vi "varint.vi"() -> ()   [LabVIEW 2011]
panel:
  out "data":i32[](array[numeric])
  out "value 2":variant
  out "value":variant
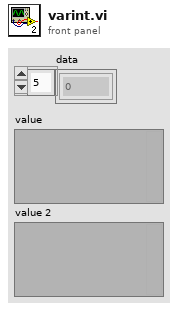
[diagram p1: front panel]
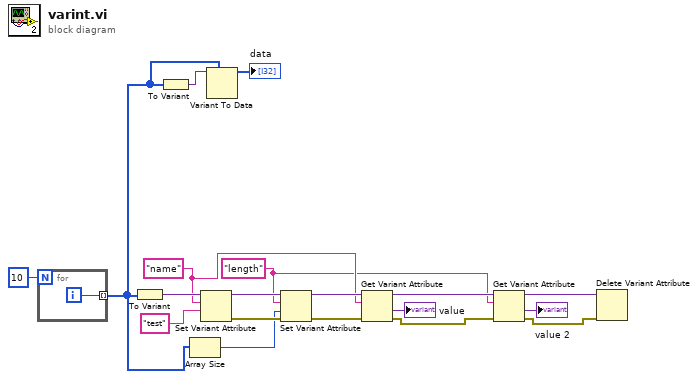
[diagram p0: block diagram]
diagram:
  w7 = "length" ("name")
  w11 = "name" ("name")
  n1 = for {
    N: 10 -> [_]
    tunnel: [w20] -> w2 mode=indexing
    i -> [w20]
  }
  n2 = To Variant(anything=w2) -> (Variant=w18:variant)
  n3 = To Variant(anything=w2) -> (Variant=w3:variant)
  n4 = Array Size(array=w2) -> (size(s)=w14:i32)
  n5 = Set Variant Attribute(Variant=w18, name=w11, value="test" ("name")) -> (Variant out=w16:variant, error out=w15:errorcluster)  [unwired: 1 in, 1 out]
  n6 = Variant To Data(type=w2, Variant=w3) -> (data=→"data":i32[])  [unwired: 1 in, 1 out]
  n7 = Set Variant Attribute(Variant=w16, name=w7, value=w14, error in=w15) -> (Variant out=w13:variant, error out=w12:errorcluster)  [unwired: 1 out]
  n8 = Get Variant Attribute(Variant=w13, name=w11, error in=w12) -> (duplicate Variant=w9:variant, value=→"value":variant, error out=w8:errorcluster)  [unwired: 1 in, 1 out]
  n9 = Get Variant Attribute(Variant=w9, name=w7, error in=w8) -> (duplicate Variant=w5:variant, value=→"value 2":variant, error out=w4:errorcluster)  [unwired: 1 in, 1 out]
  n10 = Delete Variant Attribute(4:w4, 7:w5) -> ()  [unwired: 1 in, 3 out]
